vi "PathPlanner_Trajectory_ReadCSVFile.vi"(8 "error in (no error)":errorcluster, 11 "FileName":string="trajectory.csv") -> (0 "error out":errorcluster, 3 "outTRAJECTORY":T1 {"States"."TargetHolonomicRotation"."SIN" format="%13.4f"; "States"."TargetHolonomicRotation"."COS" format="%13.4f"; "States"."TargetHolonomicRotation"."VALUE" format="%13.4f"; "States"."Heading"."SIN" format="%13.4f"; "States"."Heading"."COS" format="%13.4f"; "States"."Heading"."VALUE" format="%13.4f"; "States"."PositionMeters"."Y" format="%14.3f"; "States"."PositionMeters"."X" format="%14.3f"}, 4 "Full FIlename":string)   [LabVIEW 2019]
doc: "Create a trajectory from a CSV file. This can be used on a PC or the RoboRIO. Normally the CSV file is created as output from one of the trajectory utility programs. The file could also be created manually or by a custom written program.\n\nParameters:\n - FileName -- Name of the CSV file to read. See file name notes for additional information.\n - Error In -- Input error cluster (optional)\n\nReturns:\n - outTrajectory - Trajectory data structure cluster\n - Error out - returned error cluster\n\nNotes on use:\n -- This routine writes informational messges to the console and to the driver station log.\n\nNotes on file naming:\n -- The file name must include the extention. \".csv\" is not automatically appended to the name. \n -- The file name can be a simple file or an absolute path. If a simple file name is used the default path on the RoboRIO is: \"home:\\lvuser\\natinst\\LabVIEW Data\". On a Windows PC the default path is the LabVIEW default directory. Normally this is: “%HOMEDRIVE%%HOMEPATH%\\Documents\\LabView Data\".\n -- Filenames on the RoboRIO, which runs Linux, are case sensitive.\n\nNotes on file contents:\n -- Blank lines are ignored.\n -- Lines that begin with either #, !, or ' in the first character are considered comments and are ignored. \n -- Other lines are interpretted as comma separated data"
uses:
  TypeDef/PathPlannerTrajectory.ctl
  TypeDef/PathPlannerTrajectoryState.ctl
  <vilib>/Rock Robotics/WPI/ThirdParty/JAS_Junk/TrajLib/TypeDef/TRANSLATION2D.ctl
  <vilib>/Rock Robotics/WPI/ThirdParty/JAS_Junk/TrajLib/TypeDef/ROTATION2D.ctl
  TypeDef/PathPlannerPathConstraints.ctl
  <vilib>/Utility/error.llb/whitespace.ctl
  <vilib>/Rock Robotics/WPI/ThirdParty/JAS_Junk/TrajLib/Rotation2d_CreateAngle.vi
  <vilib>/Rock Robotics/WPI/ThirdParty/JAS_Junk/TrajLib/Util_CalcDist.vi
  <vilib>/Rock Robotics/WPI/ThirdParty/JAS_Junk/TrajLib/Trajectory_Library.lvlib
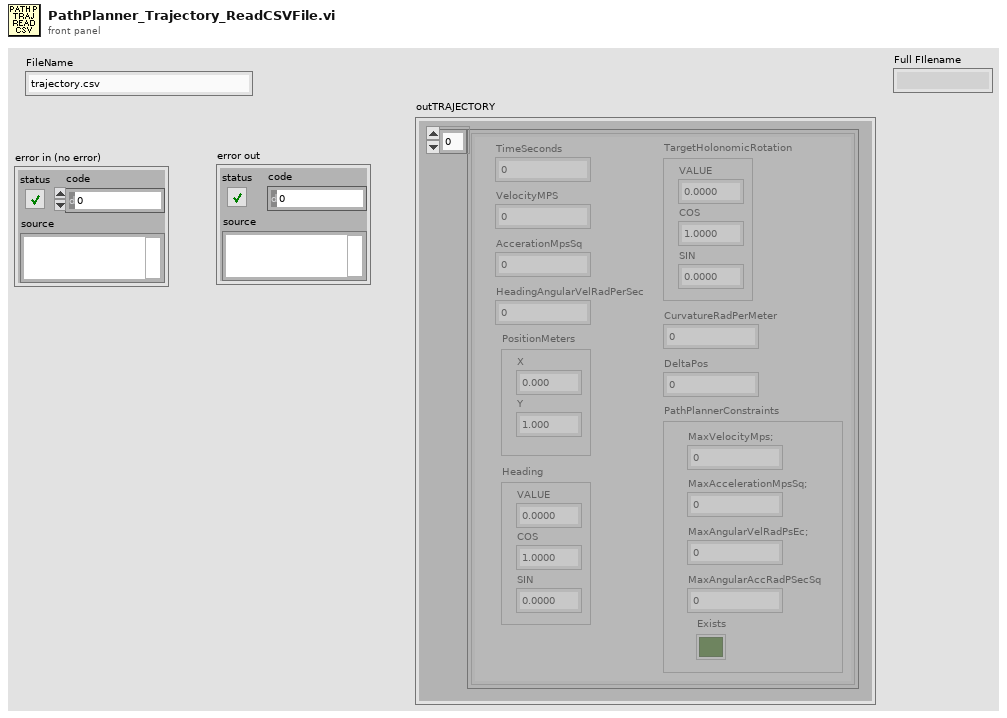
[diagram p1: front panel]
types:
  T1 = typedef "PathPlannerTrajectory.ctl" = cluster{"States":T2[]}
  T2 = typedef "PathPlannerTrajectoryState.ctl" = cluster{"TimeSeconds":dbl, "VelocityMPS":dbl, "AccerationMpsSq":dbl, "HeadingAngularVelRadPerSec":dbl, "PositionMeters":T3, "Heading":T4, "TargetHolonomicRotation":T4, "CurvatureRadPerMeter":dbl, "PathPlannerConstraints":T5, "DeltaPos":dbl}
  T3 = typedef "Trajectory_Library.lvlib/TRANSLATION2D.ctl" = cluster{"X":dbl, "Y":dbl}
  T4 = typedef "Trajectory_Library.lvlib/ROTATION2D.ctl" = cluster{"VALUE":dbl, "COS":dbl, "SIN":dbl}
  T5 = typedef "PathPlannerPathConstraints.ctl" = cluster{"MaxVelocityMps;":dbl, "MaxAccelerationMpsSq;":dbl, "MaxAngularVelRadPsEc;":dbl, "MaxAngularAccRadPSecSq":dbl, "Exists":bool}
  T6 = enum16{"open", "replace", "create", "open or create", "replace or create", "replace or create with confirmation"}
  T7 = typedef "whitespace.ctl" = u16
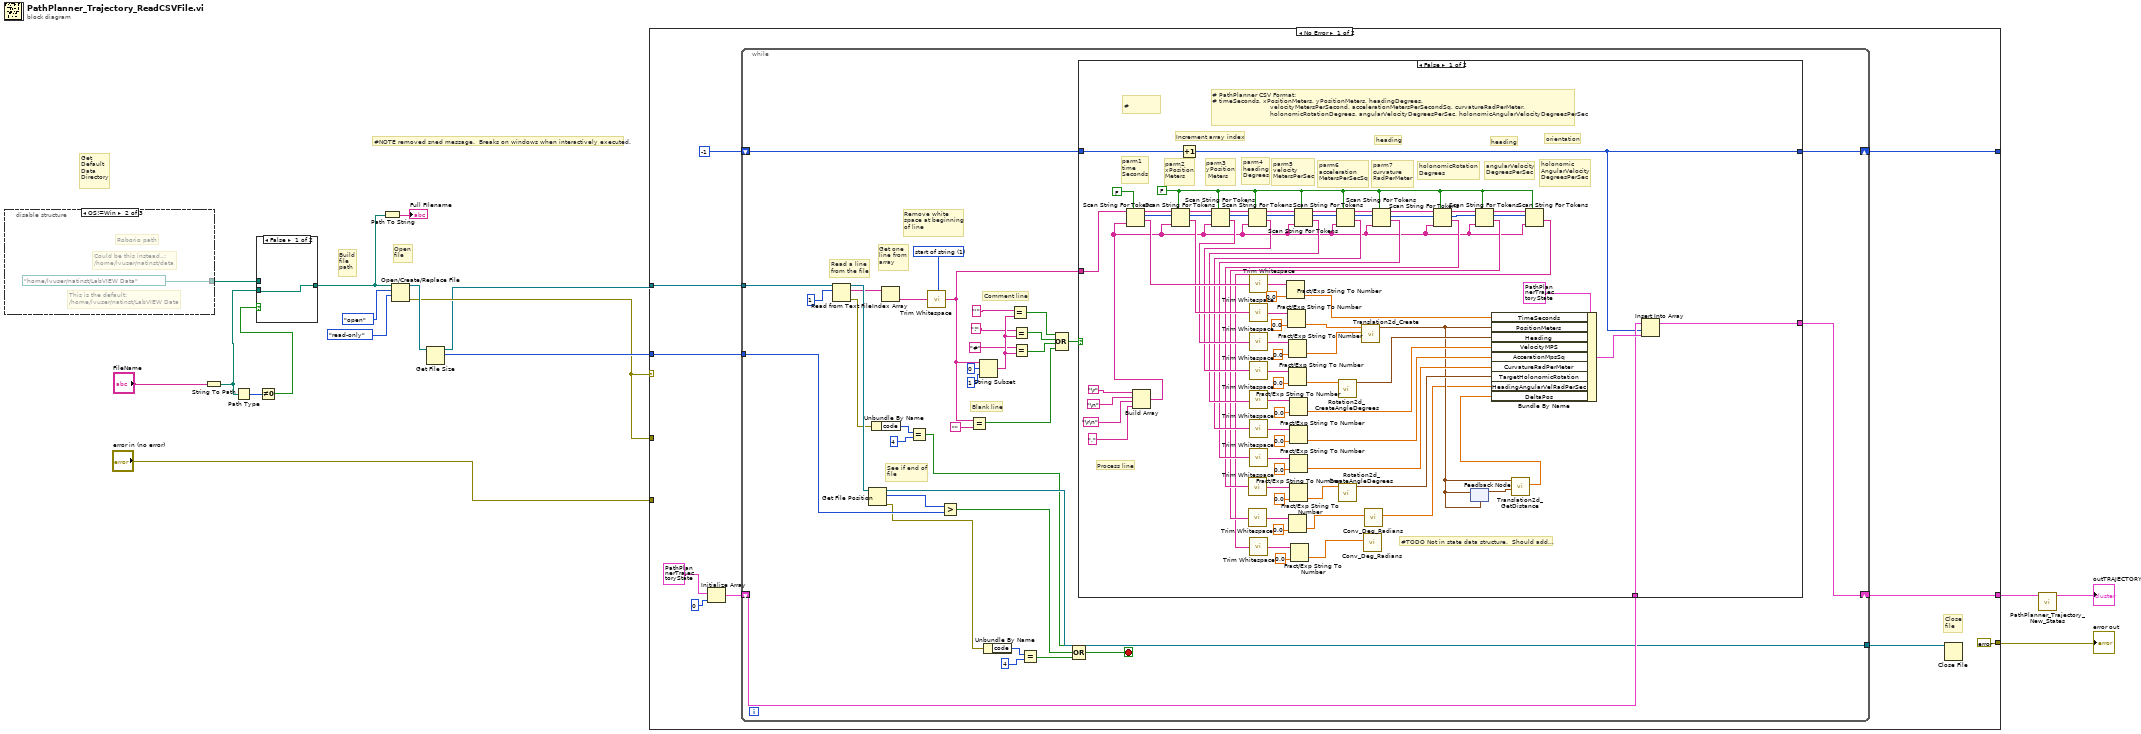
[diagram p0: block diagram]
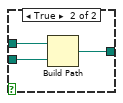
[diagram p2: hidden frame]
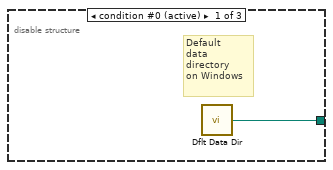
[diagram p3: hidden frame]
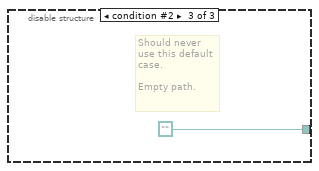
[diagram p4: hidden frame]
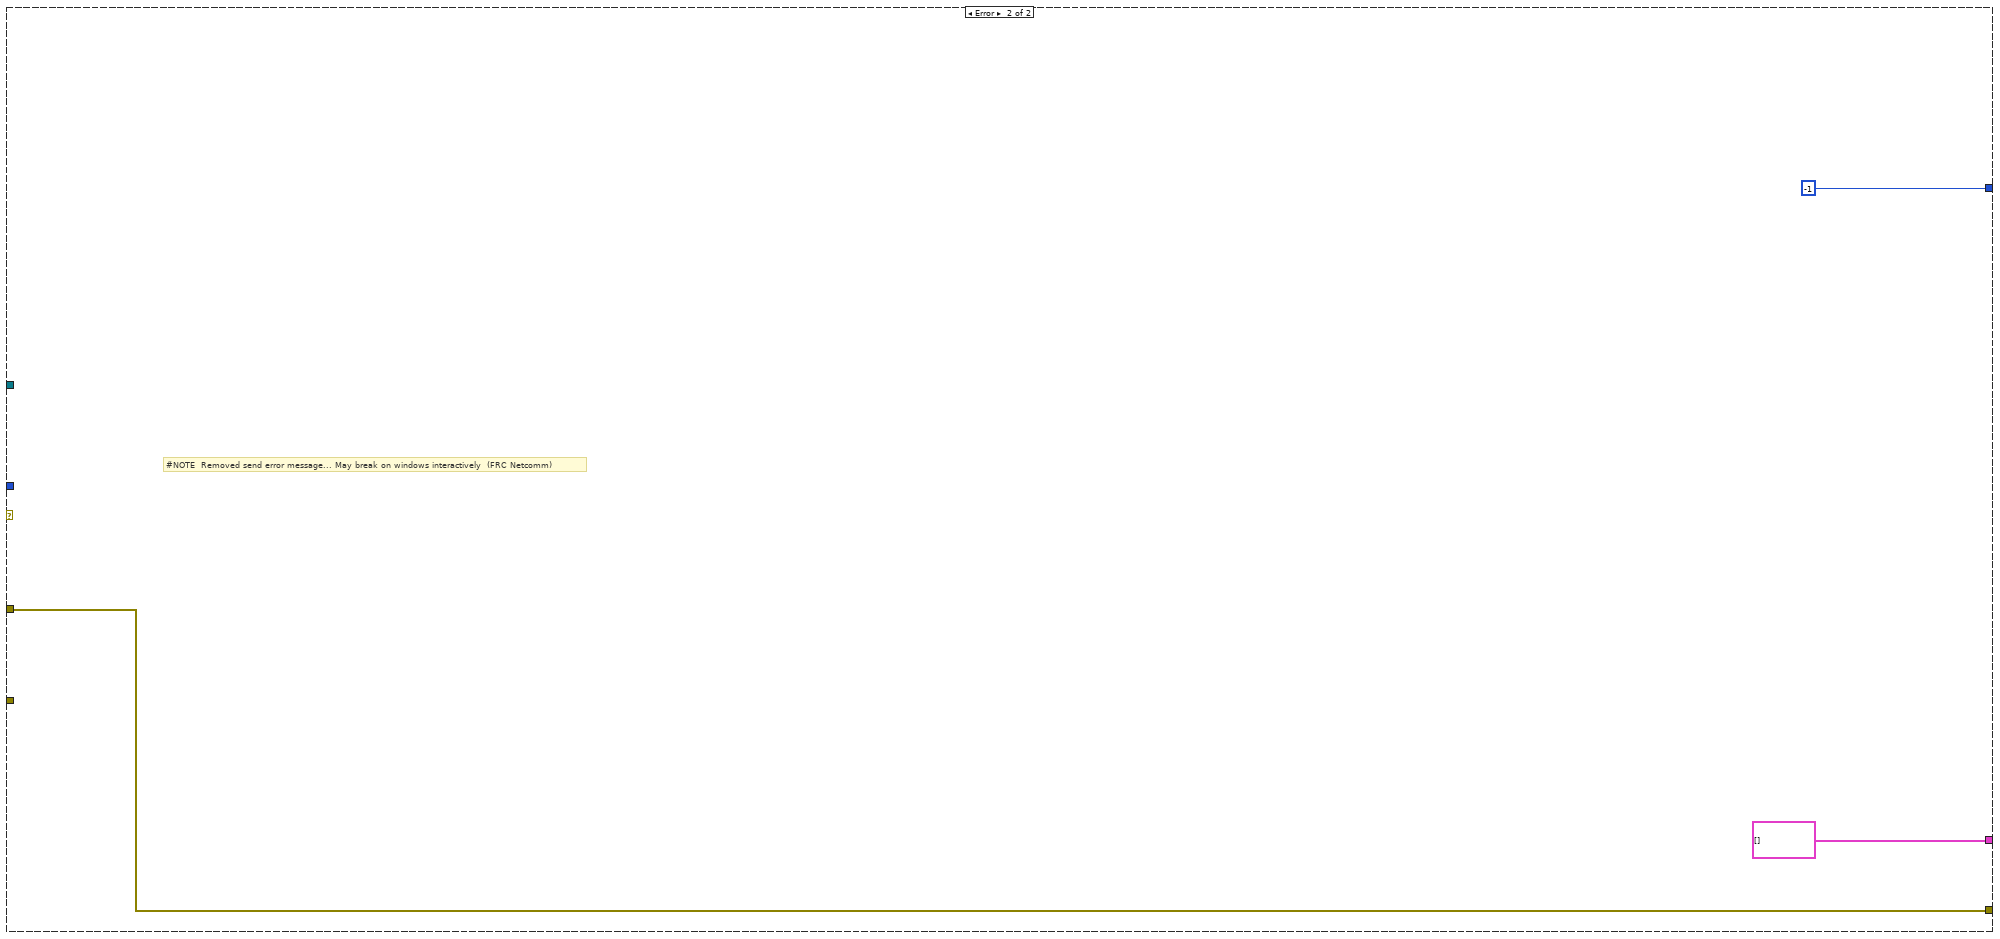
[diagram p6: hidden frame]
diagram:
  # "#NOTE removed sned message.  Breaks on windows when interactively executed."
  # "Get\nDefault\nData\nDirectory"
  # "Open\nfile"
  # "Build\nfile\npath"
  n1 = disable-structure shown="OS!=Win" {
    disable-tunnel: [w18 path "/home/lvuser/natinst/LabVIEW Data" path ""] -> w11
    frame condition #0 (active) {
      # "Default\ndata\ndirectory\non Windows"
      n2 = call <vilib>:"Dflt Data Dir.vi"() -> ("App:Default Data Directory"=w18:path)
    }
    frame condition #1 {
      # "This is the default:\n/home/lvuser/natinst/LabVIEW Data"
      # "Could be this instead..:\n/home/lvuser/natinst/data"
      # "Roborio path"
    }
    frame condition #2 {
      # "Should never\nuse this default\ncase.\n\nEmpty path."
    }
  }
  n3 = String To Path(string="FileName") -> (path=w8:path)
  n4 = Path Type(1:w8) -> (0:w7:i16)
  n5 = Not Equal To 0?(x=w7) -> (x != 0?=w6:bool)
  n6 = case shown="False" w6 {
    tunnel: [w21 w24] -> w14
    tunnel: w11 -> [_ w23]
    tunnel: w8 -> [w21 w22]
    frame False {
    }
    frame True {
      n7 = Build Path(base path=w23, name or relative path=w22) -> (appended path=w24:path)
    }
  }
  n8 = Path To String(path=w14) -> (string=→"Full FIlename":string)
  n9 = Open/Create/Replace File(file path (use dialog)=w14, operation (0:open)=T6."open", access (0:read/write)=enum16{"read/write", "read-only", "write-only"}."read-only") -> (refnum out=w15:refnum<file>, error out=w12:errorcluster)  [unwired: 3 in, 1 out]
  n10 = Get File Size(file=w15) -> (refnum out=w5:refnum<file>, size (in bytes)=w13:i64)  [unwired: 1 in, 1 out]
  n11 = case shown="No Error" w12 {
    tunnel: w5 -> [w34 _]
    tunnel: w13 -> [w32 _]
    tunnel: [w28 i16 -1] -> _
    tunnel: [w27 T2[] []] -> w2
    tunnel: w12 -> [_ w151]
    tunnel: [errorcluster {"status"=FALSE, "code"=0, "source"=""} ("error out") w151] -> w10
    tunnel: "error in (no error)" -> [_ _]
    frame No Error {
      # "Close\nfile"
      n12 = Initialize Array(T2 {"TimeSeconds"=0.0, "VelocityMPS"=0.0, "AccerationMpsSq"=0.0, "HeadingAngularVelRadPerSec"=0.0, "PositionMeters"={"X"=0.0, "Y"=1.0}, "Heading"={"VALUE"=0.0, "COS"=1.0, "SIN"=0.0}, "TargetHolonomicRotation"={"VALUE"=0.0, "COS"=1.0, "SIN"=0.0}, "CurvatureRadPerMeter"=0.0, "PathPlannerConstraints"={"MaxVelocityMps;"=0.0, "MaxAccelerationMpsSq;"=0.0, "MaxAngularVelRadPsEc;"=0.0, "MaxAngularAccRadPSecSq"=0.0, "Exists"=FALSE}, "DeltaPos"=0.0} ("PathPlannerState"), 0 ("dimension size")) -> (w29:T2[])
      n13 = while {
        tunnel: w34 -> [w70]
        tunnel: w32 -> [w66]
        tunnel: [w46] -> w31
        shift-right: [w36] -> w28
        shift-left: i16 -1 -> [w50]
        shift-right: [w35] -> w27
        shift-left: w29 -> [w48]
        stop <- w44 stop-if-true
        w65 = T7 1 items=["both", "start of string", "end of string"] ("location (both)")
        # "Comment line"
        # "Blank line"
        # "Remove white \nspace at beginning\nof line"
        # "Get one\nline from\narray"
        # "Read a line\nfrom the file"
        # "See if end of \nfile"
        n14 = Read from Text File(file (use dialog)=w70, count=1) -> (refnum out=w68:refnum<file>, text=w64:string[], error out=w47:errorcluster)  [unwired: 2 in, 1 out]
        n15 = Get File Position(7:w68) -> (0:w39:errorcluster, 2:w67:i64, 3:w46:refnum<file>)  [unwired: 1 in]
        n16 = Unbundle By Name(w47) -> ("code"=w43:i32)
        n17 = Index Array(array=w64) -> (element=w63:string)  [unwired: 1 in]
        n18 = Equal?(x=w43, y=4) -> (x = y?=w38:bool)
        n19 = call <vilib>:"Trim Whitespace.vi"("string"=w63, "location (both)"=w65) -> ("trimmed string"=w49:string)
        n20 = Greater?(x=w67, y=w66) -> (0:w45:bool)
        n21 = Equal?(x=w49, y="") -> (x = y?=w52:bool)
        n22 = String Subset(string=w49, offset (0)=0, length (rest)=1 ("length (rest)")) -> (substring=w59:string)
        n23 = Unbundle By Name(w39) -> ("code"=w41:i32)
        n24 = Equal?(x="'", y=w59) -> (x = y?=w55:bool)
        n25 = Equal?(x="!", y=w59) -> (x = y?=w54:bool)
        n26 = Equal?(x="#", y=w59) -> (x = y?=w53:bool)
        n27 = Equal?(x=w41, y=4) -> (x = y?=w37:bool)
        n28 = Compound Arithmetic op=OR(w55, w54, w53, w52) -> (w51:bool)
        n29 = Compound Arithmetic op=OR(w38, w45, w37) -> (w44:bool)
        n30 = case shown="False" w51 {
          tunnel: w50 -> [w148 w149]
          tunnel: [w113 w149] -> w36
          tunnel: w49 -> [w112 _]
          tunnel: w48 -> [w115 w150]
          tunnel: [w114 w150] -> w35
          frame False {
            w99 = FALSE ("allow empty tokens? (F)")
            # "orientation"
            # "heading"
            # "heading"
            # "#TODO Not in state data structure.  Should add..."
            # "# PathPlanner CSV Format:\n# timeSeconds, xPositionMeters, yPositionMeters, headingDegrees, \n                             velocityMetersPerSecond, accelerationMetersPerSecondSq, curvatureRadPerMeter, \n                             holonomicRotationDegrees, angularVelocityDegreesPerSec, holonomicAngularVelocityDegreesPerSec"
            # "holonomic\nAngularVelocity\nDegreesPerSec"
            # "angularVelocity\nDegreesPerSec"
            # "holonomicRotation\nDegrees"
            # "#"
            # "parm6\nacceleration\nMetersPerSecSq"
            # "parm7\ncurvature\nRadPerMeter"
            # "parm5\nvelocity\nMetersPerSec"
            # "parm4\nheading\nDegrees"
            # "parm3\nyPosition\n Meters"
            # "parm2\nxPosition\nMeters"
            # "parm1\ntime\nSeconds"
            # "Increment array index"
            # "Process line"
            n31 = Build Array("\r", "\n", "\r\n", ",") -> (w82:string[])
            n32 = Scan String For Tokens(5:FALSE ("allow empty tokens? (F)"), 6:w82, 9:w112) -> (1:w132:string, 2:w137:i32, 3:w142:string)  [unwired: 3 in, 1 out]
            n33 = Scan String For Tokens(5:w99, 6:w82, 8:w137, 9:w142) -> (1:w131:string, 2:w136:i32, 3:w141:string)  [unwired: 2 in, 1 out]
            n34 = Increment(x=w148) -> (x+1=w113:i16)
            n35 = Scan String For Tokens(5:w99, 6:w82, 8:w136, 9:w141) -> (1:w130:string, 2:w135:i32, 3:w140:string)  [unwired: 2 in, 1 out]
            n36 = Scan String For Tokens(5:w99, 6:w82, 8:w135, 9:w140) -> (1:w129:string, 2:w134:i32, 3:w139:string)  [unwired: 2 in, 1 out]
            n37 = call <vilib>:"Trim Whitespace.vi"("string"=w132) -> ("trimmed string"=w104:string)  [unwired: 1 in]
            n38 = call <vilib>:"Trim Whitespace.vi"("string"=w131) -> ("trimmed string"=w125:string)  [unwired: 1 in]
            n39 = call <vilib>:"Trim Whitespace.vi"("string"=w130) -> ("trimmed string"=w120:string)  [unwired: 1 in]
            n40 = call <vilib>:"Trim Whitespace.vi"("string"=w129) -> ("trimmed string"=w119:string)  [unwired: 1 in]
            n41 = Fract/Exp String To Number(string=w104, default (0 dbl)=0.0 ("default (0 DBL)")) -> (number=w105:dbl)  [unwired: 2 in, 1 out]
            n42 = Fract/Exp String To Number(string=w125, default (0 dbl)=0.0 ("default (0 DBL)")) -> (number=w81:dbl)  [unwired: 2 in, 1 out]
            n43 = Fract/Exp String To Number(string=w120, default (0 dbl)=0.0 ("default (0 DBL)")) -> (number=w80:dbl)  [unwired: 2 in, 1 out]
            n44 = Fract/Exp String To Number(string=w119, default (0 dbl)=0.0 ("default (0 DBL)")) -> (number=w79:dbl)  [unwired: 2 in, 1 out]
            n45 = Scan String For Tokens(5:w99, 6:w82, 8:w134, 9:w139) -> (1:w128:string, 2:w133:i32, 3:w138:string)  [unwired: 2 in, 1 out]
            n46 = call <vilib>:"Trim Whitespace.vi"("string"=w128) -> ("trimmed string"=w118:string)  [unwired: 1 in]
            n47 = Fract/Exp String To Number(string=w118, default (0 dbl)=0.0 ("default (0 DBL)")) -> (number=w102:dbl)  [unwired: 2 in, 1 out]
            n48 = Scan String For Tokens(5:w99, 6:w82, 8:w133, 9:w138) -> (1:w127:string, 2:w107:i32, 3:w108:string)  [unwired: 2 in, 1 out]
            n49 = call <vilib>:"Trim Whitespace.vi"("string"=w127) -> ("trimmed string"=w117:string)  [unwired: 1 in]
            n50 = Fract/Exp String To Number(string=w117, default (0 dbl)=0.0 ("default (0 DBL)")) -> (number=w101:dbl)  [unwired: 2 in, 1 out]
            n51 = call <vilib>:"Rotation2d_CreateAngleDegrees.vi"("Angle_Degrees"=w79) -> ("ROTATION"=w78:T4)  [unwired: 10 in]
            n52 = call <vilib>:"Translation2d_Create.vi"("Y"=w80, "X"=w81) -> ("TRANSLATION"=w74:T3)  [unwired: 9 in]
            n53 = Scan String For Tokens(5:w99, 6:w82, 8:w107, 9:w108) -> (1:w106:string, 2:w95:i32, 3:w98:string)  [unwired: 2 in, 1 out]
            n54 = call <vilib>:"Trim Whitespace.vi"("string"=w106) -> ("trimmed string"=w109:string)  [unwired: 1 in]
            n55 = Fract/Exp String To Number(string=w109, default (0 dbl)=0.0 ("default (0 DBL)")) -> (number=w100:dbl)  [unwired: 2 in, 1 out]
            n56 = Scan String For Tokens(5:w99, 6:w82, 8:w95, 9:w98) -> (1:w86:string, 2:w94:i32, 3:w97:string)  [unwired: 2 in, 1 out]
            n57 = call <vilib>:"Trim Whitespace.vi"("string"=w86) -> ("trimmed string"=w91:string)  [unwired: 1 in]
            n58 = Fract/Exp String To Number(string=w91, default (0 dbl)=0.0 ("default (0 DBL)")) -> (number=w85:dbl)  [unwired: 2 in, 1 out]
            n59 = call <vilib>:"Rotation2d_CreateAngleDegrees.vi"("Angle_Degrees"=w85) -> ("ROTATION"=w77:T4)  [unwired: 10 in]
            n60 = feedback-in #1(w74) -> ()
            n61 = feedback #1(w74) -> (w73:T3)
            n62 = Scan String For Tokens(5:w99, 6:w82, 8:w94, 9:w97) -> (1:w84:string, 2:w93:i32, 3:w96:string)  [unwired: 2 in, 1 out]
            n63 = call <vilib>:"Trim Whitespace.vi"("string"=w84) -> ("trimmed string"=w89:string)  [unwired: 1 in]
            n64 = Fract/Exp String To Number(string=w89, default (0 dbl)=0.0 ("default (0 DBL)")) -> (number=w76:dbl)  [unwired: 2 in, 1 out]
            n65 = call <vilib>:"Conv_Deg_Radians.vi"("Degress"=w76) -> ("Radians"=w71:dbl)  [unwired: 10 in]
            n66 = call <vilib>:"Translation2d_GetDistance.vi"("other Translation"=w73, "In Translation"=w74) -> ("Distance"=w72:dbl)  [unwired: 9 in]
            n67 = Bundle By Name(cluster=T2 {"TimeSeconds"=0.0, "VelocityMPS"=0.0, "AccerationMpsSq"=0.0, "HeadingAngularVelRadPerSec"=0.0, "PositionMeters"={"X"=0.0, "Y"=1.0}, "Heading"={"VALUE"=0.0, "COS"=1.0, "SIN"=0.0}, "TargetHolonomicRotation"={"VALUE"=0.0, "COS"=1.0, "SIN"=0.0}, "CurvatureRadPerMeter"=0.0, "PathPlannerConstraints"={"MaxVelocityMps;"=0.0, "MaxAccelerationMpsSq;"=0.0, "MaxAngularVelRadPsEc;"=0.0, "MaxAngularAccRadPSecSq"=0.0, "Exists"=FALSE}, "DeltaPos"=0.0} ("PathPlannerState"), "TimeSeconds"=w105, "PositionMeters"=w74, "Heading"=w78, "VelocityMPS"=w102, "AccerationMpsSq"=w101, "CurvatureRadPerMeter"=w100, "TargetHolonomicRotation"=w77, "HeadingAngularVelRadPerSec"=w71, "DeltaPos"=w72) -> (w116:T2)
            n68 = Scan String For Tokens(5:w99, 6:w82, 8:w93, 9:w96) -> (1:w83:string)  [unwired: 2 in, 3 out]
            n69 = call <vilib>:"Trim Whitespace.vi"("string"=w83) -> ("trimmed string"=w87:string)  [unwired: 1 in]
            n70 = Fract/Exp String To Number(string=w87, default (0 dbl)=0.0 ("default (0 DBL)")) -> (number=w75:dbl)  [unwired: 2 in, 1 out]
            n71 = call <vilib>:"Conv_Deg_Radians.vi"("Degress"=w75) -> ()  [unwired: 10 in, 1 out]
            n72 = Insert Into Array(array=w115, index=w113, new element=w116) -> (w114:T2[])
          }
          frame True {
            # "Comment -- ignore."
          }
        }
      }
      n73 = Close File(refnum=w31) -> ()  [unwired: 1 in, 2 out]
    }
    frame Error {
      # "#NOTE  Removed send error message... May break on windows interactively  (FRC Netcomm)"
    }
  }
  "error out" <- w10
  n74 = call "PathPlanner_Trajectory_New_States.vi"("PathPlannerStates"=w2) -> ("PathPlannerTrajectory"=→"outTRAJECTORY":T1)  [unwired: 10 in]
